vi "Inject Attribute List.vi"(6 "Attributes Ref":refnum<data-value>, 8 "error in (no error)":errorcluster, 11 "Start Spot Free Rinse in":refnum<class "Stop Spot Free Rinse.lvclass">) -> (0 "error out":errorcluster, 3 "Start Spot Free Rinse out":refnum<class "Stop Spot Free Rinse.lvclass">)   [LabVIEW 2019, in "Stop Spot Free Rinse.lvclass"]
uses:
  <vilib>/gpm_packages/@cs/Car-wash/Source/Process Steps/Stop Spot Free Rinse/Stop Spot Free Rinse.lvclass
  <vilib>/gpm_packages/@cs/lookup-table/Source/LookupTable/LookupTable.lvclass
  <vilib>/gpm_packages/@cs/lookup-table/Source/LookupTable/LookupTable.lvclass/LookupTable.ctl
  <vilib>/gpm_packages/@cs/Car-wash/Source/Process Steps/Stop Spot Free Rinse/Stop Spot Free Rinse.lvclass/Stop Spot Free Rinse.ctl
  c33ccb9b-b7c0-41f6-be99-909044508e15.vi
  <vilib>/gpm_packages/@cs/lookup-table/Source/LookupTable/Read Table Reference.vi
  c33ccb9b-b7c0-41f6-be99-909044508e15.vi/15133ace-ff91-43f0-a765-6ec4f4058dc8.vi
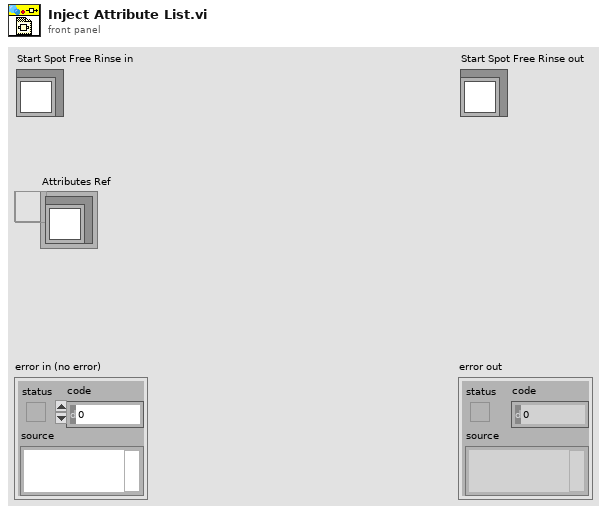
[diagram p1: front panel]
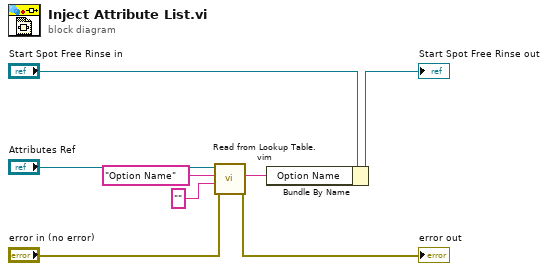
[diagram p0: block diagram]
diagram:
  n1 = call "Read from Lookup Table.vim"("error in (no error)"="error in (no error)", "Type"="", "Item Name"="Option Name", "LookupTable Reference"="Attributes Ref") -> ("error out"=→"error out":errorcluster, "Value"=w6:string)  [unwired: 4 in, 2 out]
  n2 = Bundle By Name(cluster="Start Spot Free Rinse in", "Option Name"=w6) -> (→"Start Spot Free Rinse out":refnum<class "Stop Spot Free Rinse.lvclass">)
